vi "[SubV]PDControlRight.vi"(6 "PV Old":dbl format="%#_13g", 8 "Kd":dbl, 9 "Kp":dbl, 10 "PV":dbl format="%#_13g", 11 "SP":dbl format="%#_13g") -> (2 "PV Out":dbl, 3 "Right Out":dbl)   [LabVIEW 2019]
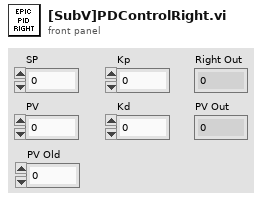
[diagram p1: front panel]
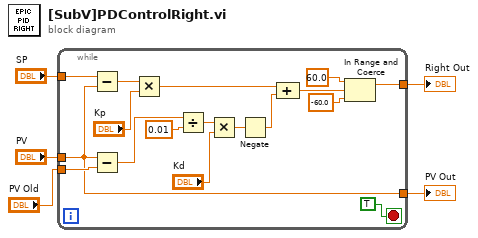
[diagram p0: block diagram]
diagram:
  n1 = while {
    tunnel: "SP" -> [w21]
    tunnel: "PV" -> [w12]
    tunnel: [w11] -> w4
    tunnel: "PV Old" -> [w19]
    tunnel: [w12] -> w1
    stop <- TRUE ("stop") stop-if-true
    n2 = Subtract(x=w21, y=w12) -> (x-y=w14:dbl)
    n3 = Subtract(x=w12, y=w19) -> (x-y=w18:dbl)
    n4 = Multiply(x=w14, y="Kp") -> (x*y=w7:dbl)
    n5 = Divide(x=w18, y=0.01) -> (x/y=w16:dbl)
    n6 = Multiply(x=w16, y="Kd") -> (x*y=w13:dbl)
    n7 = Negate(x=w13) -> (-x=w6:dbl)
    n8 = Compound Arithmetic op=ADD(w7, w6) -> (w10:dbl)
    n9 = In Range and Coerce(upper limit=60.0 ("Saturation"), x=w10, lower limit=-60.0 ("Saturation")) -> (coerced(x)=w11:dbl)  [unwired: 1 out]
  }
  "Right Out" <- w4
  "PV Out" <- w1
